vi "Snap Image.vi"(8 "error in (no error)":errorcluster, 11 "Camera Process in":refnum<class "Camera Process.lvclass">) -> (0 "error out":errorcluster, 3 "Camera Process out":refnum<class "Camera Process.lvclass">)   [LabVIEW 2022 SP3, in "Cam Process.lvlib" / "Camera Process.lvclass"]
uses:
  Camera Process.lvclass
  C:/Program Files/National Instruments/LabVIEW 2022/vi.lib/ActorFramework/Actor/Actor.lvclass
  <vilib>/ActorFramework/Actor/Actor.lvclass/Actor.ctl
  <vilib>/ActorFramework/Message Enqueuer/Message Enqueuer.lvclass/Message Enqueuer.ctl
  <vilib>/ActorFramework/Message Enqueuer/Init from Existing Queue.vi
  <vilib>/ActorFramework/Message Enqueuer/Enqueue.vi
  Camera Process Messages/Snap Image Msg/Snap Image Msg.lvclass
  C:/Program Files/National Instruments/LabVIEW 2022/vi.lib/ActorFramework/Message/Message.lvclass
  <vilib>/ActorFramework/Message Priority Queue/Priority Enqueue.vi
  <vilib>/ActorFramework/Message Enqueuer/Message Enqueuer.lvclass
  Camera Process.lvclass/Camera Process.ctl
  <vilib>/ActorFramework/Actor/Actor.lvclass
  C:/Program Files/National Instruments/LabVIEW 2022/vi.lib/MGI/Monitored Actor/Monitored Actor/Monitored Actor/Monitored Actor.lvclass
  C:/XY Stage/Camera/Camera Process/Camera Process.lvclass
  C:/XY Stage/Camera/Camera API/Camera API.lvclass
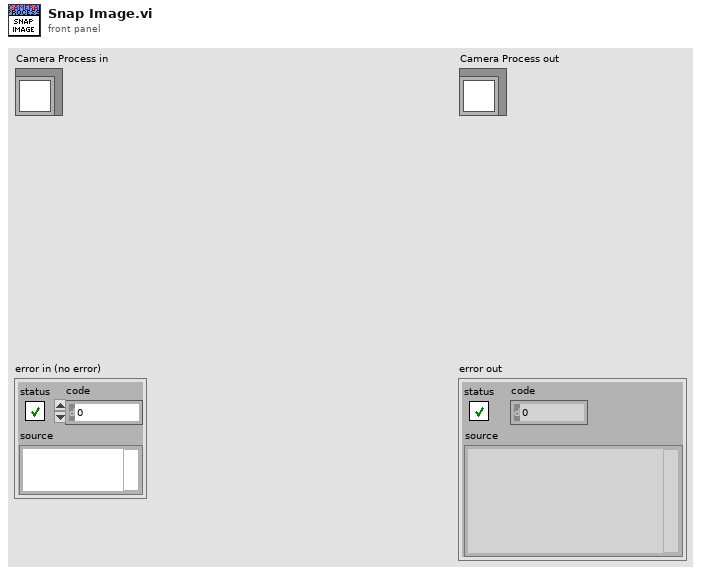
[diagram p1: front panel]
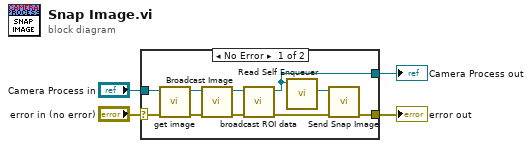
[diagram p0: block diagram]
diagram:
  n1 = case shown="No Error" "error in (no error)" {
    selector: "error in (no error)" -> [w11 w16]
    tunnel: [w13 w16] -> w3
    tunnel: [w6 w15] -> w1
    tunnel: "Camera Process in" -> [w12 w15]
    frame No Error {
      n2 = call "get image.vi"("error in (no error)"=w11, "Camera Process in"=w12) -> ("error out"=w7:errorcluster, "Camera Process out"=w10:refnum<class "Camera Process.lvclass">)  [unwired: 8 in]
      n3 = call "Broadcast Image.vi"("error in (no error)"=w7, "Camera Process in"=w10) -> ("error out"=w9:errorcluster, "Camera Process out"=w8:refnum<class "Camera Process.lvclass">)  [unwired: 8 in]
      n4 = call "broadcast ROI data.vi"("error in (no error)"=w9, "Camera Process in"=w8) -> ("error out"=w5:errorcluster, "Camera Process in 2"=w6:refnum<class "Camera Process.lvclass">)  [unwired: 8 in]
      n5 = call <vilib>:"Read Self Enqueuer.vi"("Actor"=w6) -> ("Self Enqueuer"=w14:refnum<class "Message Enqueuer.lvclass">)  [unwired: 10 in]
      n6 = call "Send Snap Image.vi"("error in (no error)"=w5, "Message Enqueuer"=w14) -> ("error out"=w13:errorcluster)  [unwired: 8 in, 1 out]
    }
    frame Error {
    }
  }
  "error out" <- w3
  "Camera Process out" <- w1
